vi "PerfAddRemove.vi"() -> (3 "Add time":dbl format="%.2p")   [LabVIEW 2024, in "RotateCircularBuffer.Tests.Perf.lvlib"]
uses:
  RotateCircularBuffer.Tests.Perf.lvlib
  RotateCircularBuffer.lvclass/RotateCircularBuffer.ctl
  TypedCircularBuffer/Type.ctl
  <vilib>/Analysis/baseanly.llb/Mean (DBL).vi
  Resize.vi
  RotateCircularBuffer.lvclass
  TypedCircularBuffer/TypedCircularBuffer.lvclass
  <vilib>/Analysis/NI_AALBase.lvlib
panel:
  out "remove time":dbl format="%.2p"
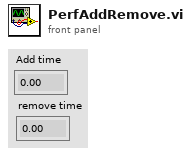
[diagram p1: front panel]
types:
  T1 = typedef "TypedCircularBuffer.lvclass/Type.ctl" = i32
  T2 = typedef "RotateCircularBuffer.lvclass/Type.ctl" = u8
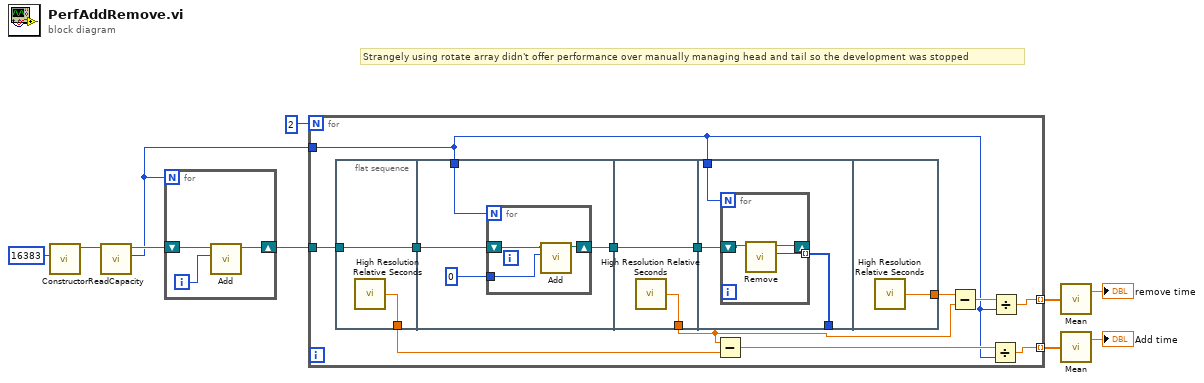
[diagram p0: block diagram]
diagram:
  # "Strangely using rotate array didn't offer performance over manually managing head and tail so the development was stopped"
  n1 = call "Constructor.vi"("Capacity"=u32 16383) -> ("TypedCircularBuffer out"=w4:refnum<class "RotateCircularBuffer.lvclass">)  [unwired: 10 in]
  n2 = call "ReadCapacity.vi"("TypedCircularBuffer in"=w4) -> ("capacity"=w1:u32, "TypedCircularBuffer out"=w3:refnum<class "RotateCircularBuffer.lvclass">)  [unwired: 9 in]
  n3 = for {
    N: w1 -> [_]
    shift-right: [w12] -> w2
    shift-left: w3 -> [w13]
    i -> [w11]
    n4 = call "Add.vi"("Element"=w11, "TypedCircularBuffer in"=w13) -> ("TypedCircularBuffer out"=w12:refnum<class "RotateCircularBuffer.lvclass">)  [unwired: 9 in]
  }
  n5 = for {
    N: 2 -> [_]
    tunnel: [w15] -> w10 mode=indexing
    tunnel: w2 -> [w24]
    tunnel: [w16] -> w6 mode=indexing
    tunnel: w1 -> [w14]
    n6 = flat-sequence {
      tunnel: w24 -> [w27]
      tunnel: [w27] -> w21
      tunnel: [w26] -> w19
      tunnel: [w30] -> w22
      tunnel: w21 -> [w31]
      tunnel: w14 -> [w28]
      tunnel: [w36] -> w20
      tunnel: [w35] -> w23
      tunnel: w22 -> [w35]
      tunnel: w23 -> [w39]
      tunnel: [w38] -> _
      tunnel: w14 -> [w37]
      tunnel: [w43] -> w25
      frame #0 {
        n7 = call <vilib>:"High Resolution Relative Seconds.vi"() -> ("relative seconds"=w26:dbl)
      }
      frame #1 {
        n8 = for {
          N: w28 -> [_]
          shift-right: [w33] -> w30
          shift-left: w31 -> [w34]
          tunnel: T1 0 ("Element") -> [w32]
          n9 = call "Add.vi"("Element"=w32, "TypedCircularBuffer in"=w34) -> ("TypedCircularBuffer out"=w33:refnum<class "RotateCircularBuffer.lvclass">)  [unwired: 9 in]
        }
      }
      frame #2 {
        n10 = call <vilib>:"High Resolution Relative Seconds.vi"() -> ("relative seconds"=w36:dbl)
      }
      frame #3 {
        n11 = for {
          N: w37 -> [_]
          shift-right: [w41] -> _
          shift-left: w39 -> [w42]
          tunnel: [w40] -> w38 mode=indexing
          n12 = call "Remove.vi"("TypedCircularBuffer in"=w42) -> ("element"=w40:T2, "TypedCircularBuffer out"=w41:refnum<class "RotateCircularBuffer.lvclass">)  [unwired: 8 in, 1 out]
        }
      }
      frame #4 {
        n13 = call <vilib>:"High Resolution Relative Seconds.vi"() -> ("relative seconds"=w43:dbl)
      }
    }
    n14 = Subtract(x=w20, y=w19) -> (x-y=w17:dbl)
    n15 = Subtract(x=w25, y=w20) -> (x-y=w18:dbl)
    n16 = Divide(x=w17, y=w14) -> (x/y=w16:dbl)
    n17 = Divide(x=w18, y=w14) -> (x/y=w15:dbl)
  }
  n18 = call-poly <vilib>:"Mean.vi"("X"=w10) -> ("mean"=→"remove time":dbl)  [unwired: 1 out]
  n19 = call-poly <vilib>:"Mean.vi"("X"=w6) -> ("mean"=→"Add time":dbl)  [unwired: 1 out]
